vi "UpdateParameterList.vi"(9 "added_string":refnum<vi>, 10 "Boolean":bool, 11 "Subst":refnum<vi>) -> ()   [LabVIEW 2016]
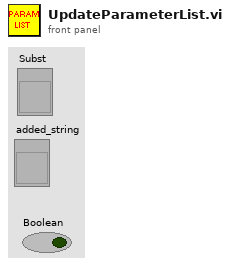
[diagram p1: front panel]
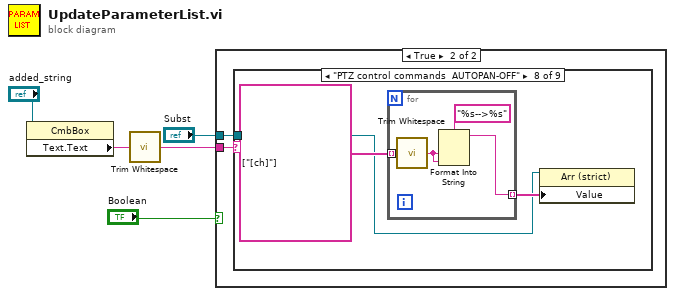
[diagram p0: block diagram]
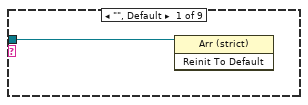
[diagram p3: hidden frame]
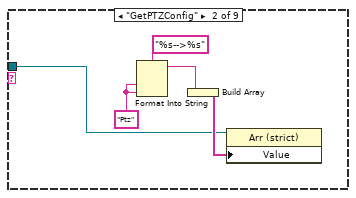
[diagram p4: hidden frame]
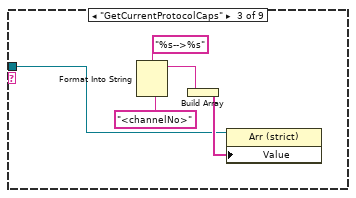
[diagram p5: hidden frame]
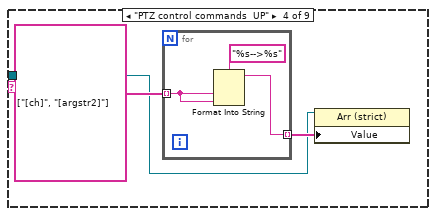
[diagram p6: hidden frame]
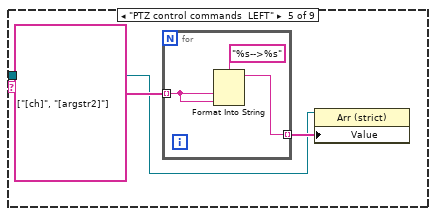
[diagram p7: hidden frame]
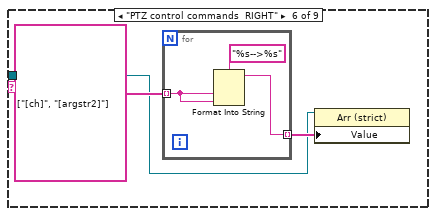
[diagram p8: hidden frame]
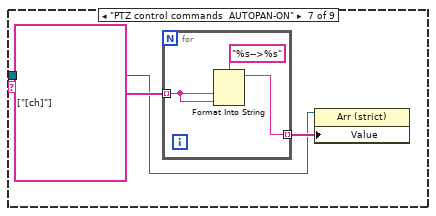
[diagram p9: hidden frame]
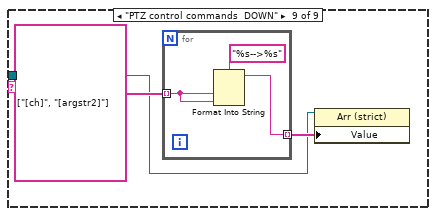
[diagram p10: hidden frame]
diagram:
  n1 = property class="CmbBox"(reference="added_string") -> ("Text.Text"=w2:string)  [unwired: 1 in, 2 out]
  n2 = call <vilib>:"Trim Whitespace.vi"("string"=w2) -> ("trimmed string"=w1:string)  [unwired: 1 in]
  n3 = case shown="True" "Boolean" {
    tunnel: w1 -> [_ w7]
    tunnel: "Subst" -> [_ w6]
    frame False {
    }
    frame True {
      n4 = case shown="\"PTZ control commands  AUTOPAN-OFF\"" w7 {
        tunnel: w6 -> [w8 w9 w14 w19 w25 w31 w37 w43 w50]
        frame "", Default {
          n5 = invoke on="Invoke Node" class="Arr (strict)" method="Reinit To Default"(reference=w8) -> ()  [unwired: 2 in, 3 out]
        }
        frame "GetPTZConfig" {
          w13 = "Ptz"
          n6 = Format Into String(format string="%s-->%s", w13, w13) -> (resulting string=w11:string)  [unwired: 2 in, 1 out]
          n7 = Build Array(w11) -> (w10:string[])
          n8 = property class="Arr (strict)"(reference=w9, "Value"=w10) -> ()  [unwired: 1 in, 2 out]
        }
        frame "GetCurrentProtocolCaps" {
          w18 = "<channelNo>"
          n9 = Format Into String(format string="%s-->%s", w18, w18) -> (resulting string=w16:string)  [unwired: 2 in, 1 out]
          n10 = Build Array(w16) -> (w15:string[])
          n11 = property class="Arr (strict)"(reference=w14, "Value"=w15) -> ()  [unwired: 1 in, 2 out]
        }
        frame "PTZ control commands  UP" {
          n12 = for {
            tunnel: string[] ["[ch]", "[argstr2]"] -> [w23] mode=indexing
            tunnel: [w22] -> w20 mode=indexing
            n13 = Format Into String(format string="%s-->%s", w23, w23) -> (resulting string=w22:string)  [unwired: 2 in, 1 out]
          }
          n14 = property class="Arr (strict)"(reference=w19, "Value"=w20) -> ()  [unwired: 1 in, 2 out]
        }
        frame "PTZ control commands  LEFT" {
          n15 = for {
            tunnel: string[] ["[ch]", "[argstr2]"] -> [w29] mode=indexing
            tunnel: [w28] -> w26 mode=indexing
            n16 = Format Into String(format string="%s-->%s", w29, w29) -> (resulting string=w28:string)  [unwired: 2 in, 1 out]
          }
          n17 = property class="Arr (strict)"(reference=w25, "Value"=w26) -> ()  [unwired: 1 in, 2 out]
        }
        frame "PTZ control commands  RIGHT" {
          n18 = for {
            tunnel: string[] ["[ch]", "[argstr2]"] -> [w35] mode=indexing
            tunnel: [w34] -> w32 mode=indexing
            n19 = Format Into String(format string="%s-->%s", w35, w35) -> (resulting string=w34:string)  [unwired: 2 in, 1 out]
          }
          n20 = property class="Arr (strict)"(reference=w31, "Value"=w32) -> ()  [unwired: 1 in, 2 out]
        }
        frame "PTZ control commands  AUTOPAN-ON" {
          n21 = for {
            tunnel: string[] ["[ch]"] -> [w41] mode=indexing
            tunnel: [w40] -> w38 mode=indexing
            n22 = Format Into String(format string="%s-->%s", w41, w41) -> (resulting string=w40:string)  [unwired: 2 in, 1 out]
          }
          n23 = property class="Arr (strict)"(reference=w37, "Value"=w38) -> ()  [unwired: 1 in, 2 out]
        }
        frame "PTZ control commands  AUTOPAN-OFF" {
          n24 = for {
            tunnel: string[] ["[ch]"] -> [w48] mode=indexing
            tunnel: [w47] -> w44 mode=indexing
            n25 = call <vilib>:"Trim Whitespace.vi"("string"=w48) -> ("trimmed string"=w46:string)  [unwired: 1 in]
            n26 = Format Into String(format string="%s-->%s", w46, w46) -> (resulting string=w47:string)  [unwired: 2 in, 1 out]
          }
          n27 = property class="Arr (strict)"(reference=w43, "Value"=w44) -> ()  [unwired: 1 in, 2 out]
        }
        frame "PTZ control commands  DOWN" {
          n28 = for {
            tunnel: string[] ["[ch]", "[argstr2]"] -> [w54] mode=indexing
            tunnel: [w53] -> w51 mode=indexing
            n29 = Format Into String(format string="%s-->%s", w54, w54) -> (resulting string=w53:string)  [unwired: 2 in, 1 out]
          }
          n30 = property class="Arr (strict)"(reference=w50, "Value"=w51) -> ()  [unwired: 1 in, 2 out]
        }
      }
    }
  }
